vi "Send WebSocket Data Handler.vi"(0 "Message Enqueuer":refnum<class "Message Enqueuer.lvclass">, 1 "Message Priority (Normal)":T2=enum."Normal", 2 "Message Type":refnum<class "WebSocket Connection Handler Msg.lvclass">, 5 "Connection Event":T1, 7 "Peer ID":string, 9 "Data":string, 11 "error in (no error)":errorcluster, 12 "Connection Enqueuer":refnum<class "Message Enqueuer.lvclass">) -> (4 "Message Enqueuer out":refnum<class "Message Enqueuer.lvclass">, 15 "error out":errorcluster)   [LabVIEW 2016, in "WebSocket Actors.lvlib" / "WebSocket Connection Handler Msg.lvclass"]
doc: "This VI sends the message to an actor."
uses:
  WebSocket Connection Handler Msg.lvclass
  <vilib>/ActorFramework/Message Enqueuer/Message Enqueuer.lvclass
  <vilib>/ActorFramework/Message Enqueuer/Message Priority.ctl
  C:/Program Files (x86)/National Instruments/LabVIEW 2016/vi.lib/ActorFramework/Message/Message.lvclass
  properties/Connection Event.ctl
  WebSocket Connection Handler Msg.lvclass/WebSocket Connection Handler Msg.ctl
  <vilib>/ActorFramework/Message Enqueuer/Message Enqueuer.lvclass/Message Enqueuer.ctl
  <vilib>/ActorFramework/Message Priority Queue/Priority Enqueue.vi
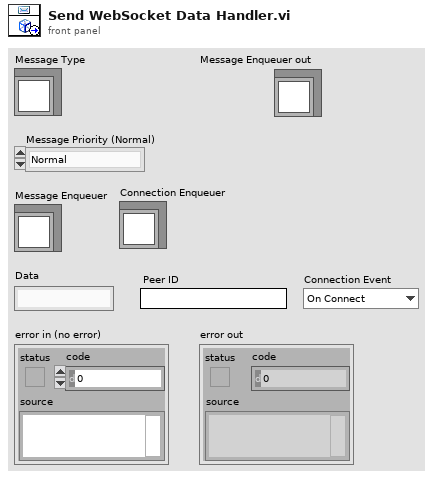
[diagram p1: front panel]
types:
  T1 = typedef "WebSocket Actors.lvlib/WebSocket Connection Handler Msg.lvclass/Connection Event.ctl" = enum16{"On Connect", "On Message", "On Close", "On Drop"}
  T2 = typedef "Actor Framework.lvlib/Message Enqueuer.lvclass/Message Priority.ctl" = enum16{"Low", "Normal", "High"}
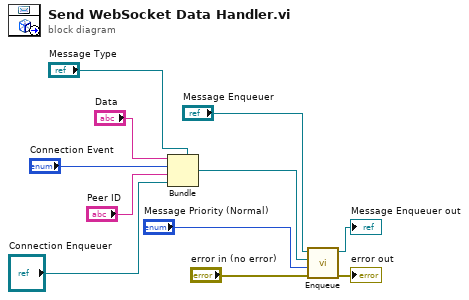
[diagram p0: block diagram]
diagram:
  n1 = Bundle(cluster="Message Type", "Data", "Connection Event", "Peer ID", "Connection Enqueuer") -> (w7:refnum<class "WebSocket Connection Handler Msg.lvclass">)
  n2 = call <vilib>:"Enqueue.vi"("error in (no error)"="error in (no error)", "Message Priority (Normal)"="Message Priority (Normal)", "Message"=w7, "Message Enqueuer in"="Message Enqueuer") -> ("error out"=→"error out":errorcluster, "Message Enqueuer out"=→"Message Enqueuer out":refnum<class "Message Enqueuer.lvclass">)  [unwired: 6 in]
